vi "Lab3_ASK_2.vi"() -> ()   [LabVIEW 2019]
uses:
  <vilib>/addons/Modulation/Analog/support/mod_Set Error Source.vi
  <vilib>/addons/Modulation/Digital/Support/Common/Validators/mod_AWGN Validate.vi
  <vilib>/addons/Modulation/Digital/Impairments/subVIs/mod_createSeeds.vi
  <vilib>/addons/Modulation/Digital/Support/Common/Validators/mod_Validate Samples Per Symbol.vi
  <vilib>/addons/Modulation/Analog/support/Validators/mod_Validate Complex Waveform.vi
  <vilib>/addons/Modulation/Analog/support/Validators/mod_WFErrorHandler.vi
  <vilib>/addons/Modulation/Digital/General/MT Generate ASK system parameters (M).vi
  <vilib>/addons/Modulation/Digital/Support/Common/Validators/mod_Generate Filter Coefficients Validate.vi
  <vilib>/addons/Modulation/Digital/General/subVIs/mod_Generate Filter Coefficients.vi
  <vilib>/addons/Modulation/Digital/General/subVIs/mod_Generate Bits PN Sequence.vi
  <vilib>/Analysis/1siggen.llb/Gaussian White Noise (obs 90).vi
  <vilib>/addons/Modulation/Analog/MT Upconvert Baseband (Real).vi
  <vilib>/express/express analysis/Spectral/Block/exnSpectralBlock spectral measurements RMS poly.vi
  <vilib>/express/express analysis/Spectral/Block/exnSpectralBlock spectral measurements RMS DDT.vi
  <vilib>/express/express analysis/Spectral/XNode/ExpressSpectralMeasurementsBlockNode.xnode
  <vilib>/addons/Modulation/niDMT.lvlib
  <vilib>/addons/Modulation/niAMT.lvlib
panel:
  in  "Tab Control":T1(tab)
  out "Waveform Graph":cluster{"t0":dbl, "dt":dbl, "Y":dbl[]}(graph)
  out "Upconverted Wave":waveform(dbl)(graph)
  out "ASK Constellation":T2(graph)
  out "Waveform Graph 2":dynamicdata(graph)
  in  "Add Bit Padding":bool
  in  "InputStrig":string
  out "Match Found?":bool
  out "Demodulated String":string
  in  "Reset":bool=TRUE
  in  "Symbol Rate(HZ)":dbl format="%#_2p"
  in  "Carrier Freq(HZ)":dbl format="%#_2p"
  in  "pulse shaping filter":T3(ring)
  in  "M-ASK":u16(ring) items=["2"=2, "4"=4, "8"=8, "16"=16]
  in  "Eb/No(dB)":dbl
  in  "stop":bool
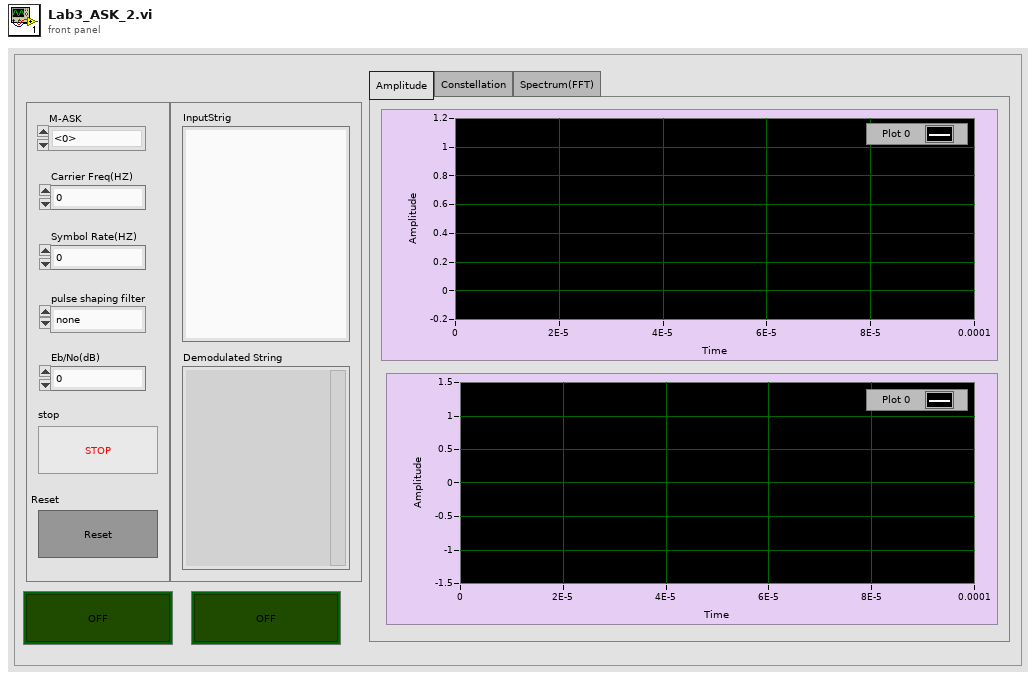
[diagram p1: front panel]
types:
  T1 = enum32{"Amplitude", "Constellation", "Spectrum(FFT)"}
  T2 = cluster{"Decimated Array":dbl[], "Decimated Array":dbl[]}[]
  T3 = enum16{"none", "Raised Cosine", "Root Raised Cos", "Gaussian"}
  T4 = enum16{"FSK", "PSK", "QAM", "MSK", "PAM", "ASK", "CPM"}
  T5 = cluster{"averaging mode":u16, "weighting mode":u16, "number of averages":u32}
  T6 = cluster{"dB On (F)":bool, "unwrap phase (F)":bool, "convert to degree (F)":bool}
  T7 = cluster{"samples per symbol (16)":i32, "symbol map":cdb[]}
  T8 = typedef "niAMT.lvlib/Complex Data Waveform.ctl" = cluster{"t0":dbl, "dt":dbl, "Y":cdb[]}
  T9 = cluster{"constellation":dbl[], "oversampled data":dbl[]}[]
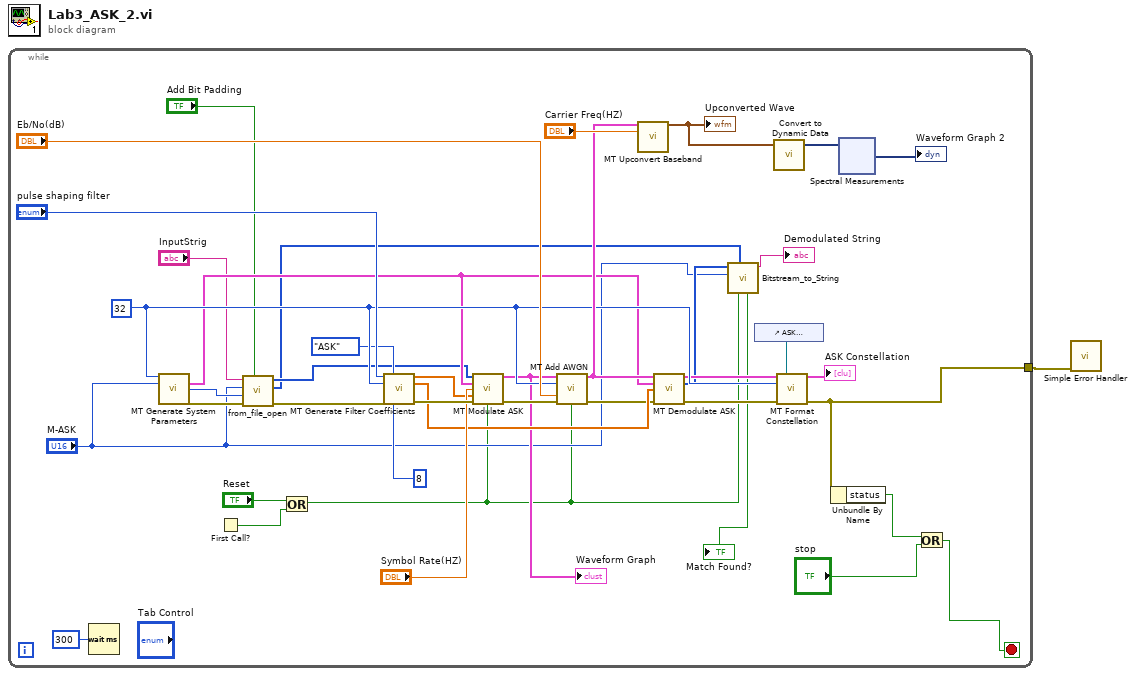
[diagram p0: block diagram]
diagram:
  n1 = while {
    tunnel: [w25] -> w1
    stop <- w22 stop-if-true
    w29 = 32 ("samples per symbol (16)")
    n2 = Wait (ms)(milliseconds to wait=u32 300) -> ()  [unwired: 1 out]
    n3 = call-poly <vilib>:"MT Generate System Parameters.vi"("samples per symbol (16)"=w29, "M-ASK (2)"="M-ASK") -> ("ASK system parameters"=w28:T7, "bits per symbol"=w18:i32, "error out"=w19:errorcluster)  [unwired: 11 in]
    n4 = First Call?() -> (First Call?: T/F=w14:bool)
    n5 = call "from_file_open.vi"("Add Bit Padding"="Add Bit Padding", "error in (no error)"=w19, "Guard Bits to Add"=w18, "M-ary (16)"="M-ASK", "InputStrig"="InputStrig") -> ("error out"=w15:errorcluster, "Character Array"=w7:u8[], "Bitstream (with Guard Bits)"=w8:i8[])  [unwired: 1 in, 2 out]
    n6 = Or(x="Reset", y=w14) -> (x .or. y?=w4:bool)
    n7 = call <vilib>:"MT Generate Filter Coefficients.vi"("pulse shaping filter (none)"="pulse shaping filter", "modulation type"=T4."ASK", "pulse shaping samples per symbol (16)"=w29, "error in (no error)"=w15, "filter length (symbols)"=8) -> ("pulse shaping filter coefficients"=w31:dbl[], "matched filter coefficients"=w32:dbl[], "error out"=w36:errorcluster)  [unwired: 8 in]
    n8 = call <vilib>:"MT Modulate ASK.vi"("input bit stream"=w8, "ASK system parameters"=w28, "symbol rate (Hz)"="Symbol Rate(HZ)", "pulse shaping filter coefficients"=w31, "error in (no error)"=w36, "reset? (T)"=w4) -> ("output complex waveform"=w26:T8, "error out"=w35:errorcluster)  [unwired: 7 in, 1 out]
    "Waveform Graph" <- w26
    n9 = call <vilib>:"MT Add AWGN.vi"("input complex waveform"=w26, "samples per symbol (16)"=w29, "Eb/N0 (10 dB)"="Eb/No(dB)", "error in (no error)"=w35, "reset? (T)"=w4) -> ("output complex waveform"=w33:T8, "error out"=w16:errorcluster)  [unwired: 8 in, 1 out]
    n10 = call-poly <vilib>:"MT Upconvert Baseband.vi"("baseband waveform (complex)"=w33, "carrier frequency (Hz)"="Carrier Freq(HZ)") -> ("passband waveform"=w9:waveform(dbl))  [unwired: 12 in, 1 out]
    "Upconverted Wave" <- w9
    n11 = call <vilib>:"MT Demodulate ASK.vi"("input complex waveform"=w33, "ASK system parameters"=w28, "matched filter coefficients"=w32, "error in (no error)"=w16) -> ("recovered complex waveform"=w21:T8, "output bit stream"=w6:i8[], "error out"=w17:errorcluster)  [unwired: 7 in, 2 out]
    n12 = call "Bitstream_to_String.vi"("Reset"=w4, "Character Array"=w7, "M-ary (16)"="M-ASK", "Bit Array"=w6) -> ("Demodulated String"=→"Demodulated String":string, "Match Found?"=→"Match Found?":bool)  [unwired: 2 in, 4 out]
    n13 = control-ref of="ASK Constellation"() -> (w41:refnum<vi>)
    n14 = call "Convert to Dynamic Data"("Waveform"=w9) -> ("Dynamic Data Type"=w11:dynamicdata)  [unwired: 3 in]
    n15 = call <vilib>:"MT Format Constellation.vi"("waveform"=w21, "constellation reference"=w41, "samples per symbol"=w29, "error in (no error)"=w17) -> ("constellation graph"=→"ASK Constellation":T9, "error out"=w25:errorcluster)  [unwired: 1 in, 9 out]
    n16 = Unbundle By Name(w25) -> ("status"=w24:bool)
    n17 = xnode ("Spectral Measurements")("Signals"=w11) -> ("FFT - (RMS)"=→"Waveform Graph 2":dynamicdata)  [unwired: 1 in, 2 out]
    n18 = Or(x=w24, y="stop") -> (x .or. y?=w22:bool)
  }
  n19 = call <vilib>:"Simple Error Handler.vi"("error in (no error)"=w1) -> ()  [unwired: 4 in, 5 out]
